vi "FRCts20_Backend_Test_Team.vi"() -> ()   [LabVIEW 2013, in "FRCts20_Backend_TestCode.lvlib"]
uses:
  FRCts20_Backend_TestCode.lvlib
  FRCts20_Backend_API/FRCts20_Backend_API_Command_App.ctl
  FRCts20_Backend_API/FRCts20_Backend_API_TeamRoot.ctl
  FRCts20_Backend_API/FRCts20_Backend_API_SW.ctl
  FRCts20_Backend_API/FRCts20_Backend_API_Team.ctl
  FRCts20_Backend_API/FRCts20_Backend_API_Status.ctl
  FRCts20_Backend_API/FRCts20_Backend_API_Application.vi
  FRCts20_Backend_API/FRCts20_Backend_API.lvlib
  FRCts20_Backend_Engine.lvlib
panel:
  out "Get Root Pass/Fail":bool
  out "Get Root":u32
  out "Get Pass/Fail":bool
  out "error out":errorcluster
  out "Del Pass/Fail":bool
  out "GetDel":u32
  out "Del":u32
  out "GetPut":u32
  out "Put":u32
  out "Put Pass/Fail":bool
  out "Post Pass/Fail":bool
  out "GetRootPost":u32
  out "post":u32
  out "Get":u32
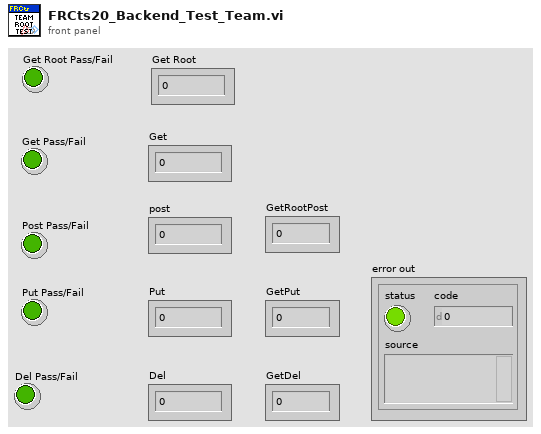
[diagram p1: front panel]
types:
  T1 = typedef "FRCts20_Backend_API.lvlib/FRCts20_Backend_API_Team.ctl" = cluster{"Team Index":u32, "Team Number":u32, "Team Name":string, "Short Team Name":string, "Nick Name":string, "Robot Name":string, "City":string, "State":string, "Country":string, "Rookie Year":u32, "SWType":T2, "CAN":bool, "Vision":bool, "Kinect":bool, "Tags":string, "Avatar":string, "Request Array":cluster{"Request Index":u32, "Description":string, "Status":T3, "Open Date":timestamp, "Last Update":timestamp, "Close Date":timestamp}[], "Events Attending":cluster{"EventIndex":dbl, "EventName":string, "IsLive":bool}[], "APIReturn":string}
  T2 = typedef "FRCts20_Backend_API.lvlib/FRCts20_Backend_API_SW.ctl" = string
  T3 = typedef "FRCts20_Backend_API.lvlib/FRCts20_Backend_API_Status.ctl" = enum16{"Open", "In Work", "Closed"}
  T4 = typedef "FRCts20_Backend_API.lvlib/FRCts20_Backend_API_TeamRoot.ctl" = cluster{"Teams":cluster{"Team Index":u32, "Team Number":u32, "Team Name":string, "Short Team Name":string, "Nick Name":string, "Robot Name":string, "City":string, "State":string, "Country":string, "Rookie Year":u32, "SWType":T2, "CAN":bool, "Vision":bool, "Kinect":bool, "Tags":string, "Avatar":string, "Events":cluster{"EventIndex":u32, "EventName":string, "IsLive":bool}[]}[], "APIReturn":string}
  T5 = typedef "FRCts20_Backend_API.lvlib/FRCts20_Backend_API_Command_App.ctl" = string
  T6 = cluster{"Team Index":u32, "Team Number":u32, "Team Name":string, "Short Team Name":string, "Nick Name":string, "Robot Name":string, "City":string, "State":string, "Country":string, "Rookie Year":u32, "SWType":T2, "CAN":bool, "Vision":bool, "Kinect":bool, "Tags":string, "Avatar":string, "Events":cluster{"EventIndex":u32, "EventName":string, "IsLive":bool}[]}[]
  T7 = cluster{"Team Index":u32, "Team Number":u32, "Team Name":string, "Short Team Name":string, "Nick Name":string, "Robot Name":string, "City":string, "State":string, "Country":string, "Rookie Year":u32, "SWType":T2, "CAN":bool, "Vision":bool, "Kinect":bool, "Tags":string, "Avatar":string, "Events":cluster{"EventIndex":u32, "EventName":string, "IsLive":bool}[]}
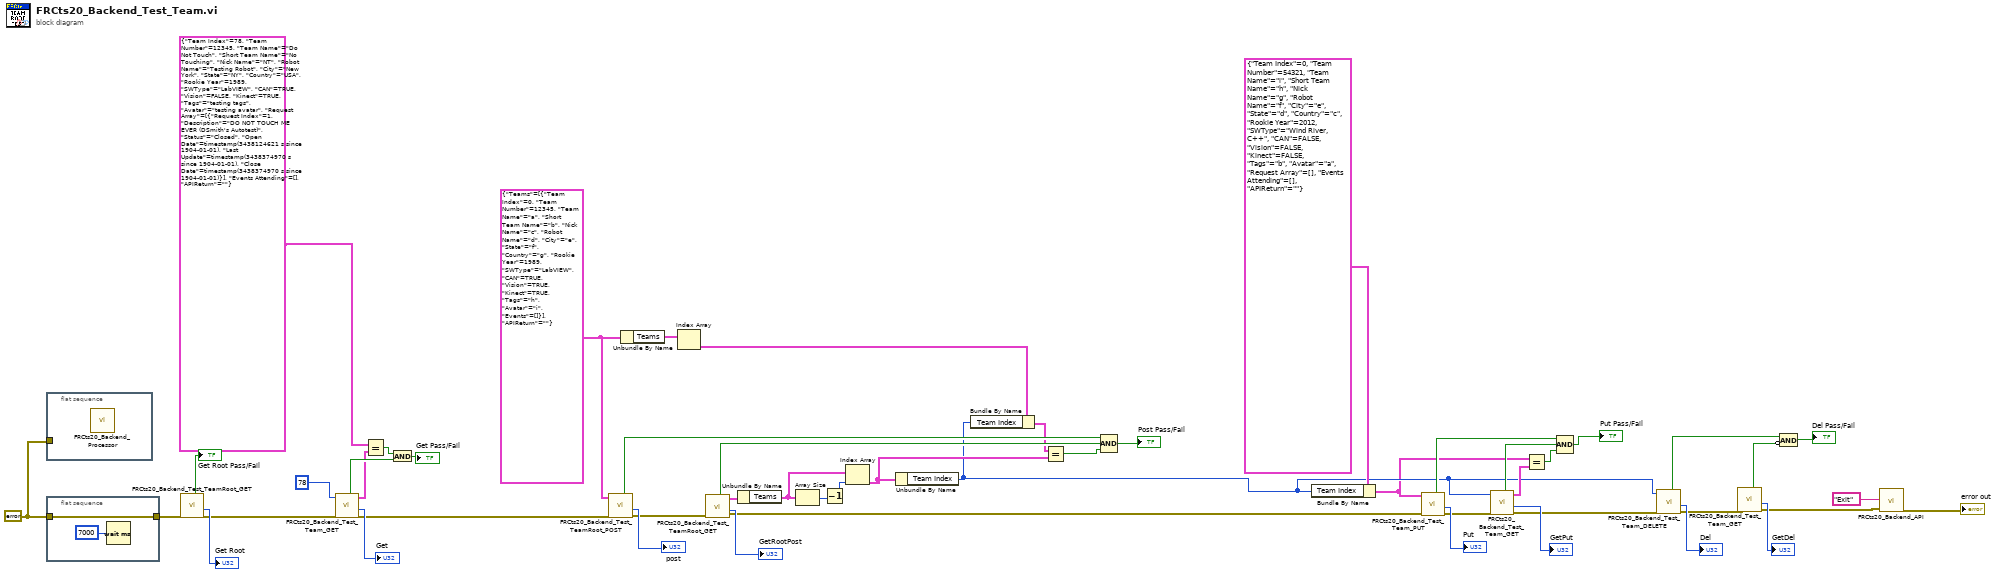
[diagram p0: block diagram]
diagram:
  w11 = T4 {"Teams"=[{"Team Index"=0, "Team Number"=12345, "Team Name"="a", "Short Team Name"="b", "Nick Name"="c", "Robot Name"="d", "City"="e", "State"="f", "Country"="g", "Rookie Year"=1989, "SWType"="LabVIEW", "CAN"=TRUE, "Vision"=TRUE, "Kinect"=TRUE, "Tags"="h", "Avatar"="i", "Events"=[]}], "APIReturn"=""} ("TeamRoot In")
  w50 = errorcluster {"status"=FALSE, "code"=0, "source"=""} ("error constant")
  n1 = flat-sequence {
    tunnel: w50 -> [_]
    frame #0 {
      n2 = call "FRCts20_Backend_Processor.vi"() -> ()  [unwired: 12 in]
    }
  }
  n3 = flat-sequence {
    tunnel: w50 -> [w52]
    tunnel: [w52] -> w48
    frame #0 {
      n4 = Wait (ms)(milliseconds to wait=u32 7000) -> ()  [unwired: 1 out]
    }
  }
  n5 = call "FRCts20_Backend_Test_TeamRoot_GET.vi"("error in (no error)"=w48) -> ("error out"=w45:errorcluster, "Time (ms)"=→"Get Root":u32, "Success"=→"Get Root Pass/Fail":bool)  [unwired: 6 in, 2 out]
  n6 = call "FRCts20_Backend_Test_Team_GET.vi"("error in (no error)"=w45, "Team Index"=u32 78) -> ("error out"=w42:errorcluster, "Time (ms)"=→"Get":u32, "Team Out"=w16:T1, "Success"=w18:bool)  [unwired: 5 in, 1 out]
  n7 = Equal?(x=T1 {"Team Index"=78, "Team Number"=12345, "Team Name"="Do Not Touch", "Short Team Name"="No Touching", "Nick Name"="NT", "Robot Name"="Testing Robot", "City"="New York", "State"="NY", "Country"="USA", "Rookie Year"=1989, "SWType"="LabVIEW", "CAN"=TRUE, "Vision"=FALSE, "Kinect"=TRUE, "Tags"="testing tags", "Avatar"="testing avatar", "Request Array"=[{"Request Index"=1, "Description"="DO NOT TOUCH ME EVER (DSmith's Autotest)", "Status"=enum."Closed", "Open Date"=timestamp(3438124621 s since 1904-01-01), "Last Update"=timestamp(3438374970 s since 1904-01-01), "Close Date"=timestamp(3438374970 s since 1904-01-01)}], "Events Attending"=[], "APIReturn"=""} ("Team Out"), y=w16) -> (x = y?=w17:bool)
  n8 = And(x=w17, y=w18) -> (x .and. y?=→"Get Pass/Fail":bool)
  n9 = call "FRCts20_Backend_Test_TeamRoot_POST.vi"("error in (no error)"=w42, "TeamRoot In"=w11) -> ("error out"=w40:errorcluster, "Time (ms)"=→"post":u32, "Success"=w29:bool)  [unwired: 5 in, 2 out]
  n10 = Unbundle By Name(w11) -> ("Teams"=w10:T6)
  n11 = Index Array(array=w10) -> (element=w8:T7)  [unwired: 1 in]
  n12 = call "FRCts20_Backend_Test_TeamRoot_GET.vi"("error in (no error)"=w40) -> ("error out"=w38:errorcluster, "Time (ms)"=→"GetRootPost":u32, "Team Out"=w15:T4, "Success"=w28:bool)  [unwired: 6 in, 1 out]
  n13 = Unbundle By Name(w15) -> ("Teams"=w12:T6)
  n14 = Array Size(array=w12) -> (size(s)=w14:i32)
  n15 = Decrement(x=w14) -> (x-1=w13:i32)
  n16 = Index Array(array=w12, index=w13) -> (element=w9:T7)
  n17 = Unbundle By Name(w9) -> ("Team Index"=w7:u32)
  n18 = Bundle By Name(cluster=w8, "Team Index"=w7) -> (w6:T7)
  n19 = Equal?(x=w6, y=w9) -> (x = y?=w27:bool)
  n20 = Compound Arithmetic op=AND(w29, w28, w27) -> (→"Post Pass/Fail":bool)
  n21 = Bundle By Name(cluster=T1 {"Team Index"=0, "Team Number"=54321, "Team Name"="i", "Short Team Name"="h", "Nick Name"="g", "Robot Name"="f", "City"="e", "State"="d", "Country"="c", "Rookie Year"=2012, "SWType"="Wind River, C++", "CAN"=FALSE, "Vision"=FALSE, "Kinect"=FALSE, "Tags"="b", "Avatar"="a", "Request Array"=[], "Events Attending"=[], "APIReturn"=""} ("Team In"), "Team Index"=w7) -> (w5:T1)
  n22 = call "FRCts20_Backend_Test_Team_PUT.vi"("error in (no error)"=w38, "Team In"=w5) -> ("error out"=w36:errorcluster, "Time (ms)"=→"Put":u32, "Success"=w24:bool)  [unwired: 5 in, 2 out]
  n23 = call "FRCts20_Backend_Test_Team_GET.vi"("error in (no error)"=w36, "Team Index"=w7) -> ("error out"=w34:errorcluster, "Time (ms)"=→"GetPut":u32, "Team Out"=w21:T1, "Success"=w23:bool)  [unwired: 5 in, 1 out]
  n24 = Equal?(x=w5, y=w21) -> (x = y?=w22:bool)
  n25 = Compound Arithmetic op=AND(w24, w23, w22) -> (→"Put Pass/Fail":bool)
  n26 = call "FRCts20_Backend_Test_Team_DELETE.vi"("error in (no error)"=w34, "Team Index"=w7) -> ("error out"=w32:errorcluster, "Time (ms)"=→"Del":u32, "Success"=w4:bool)  [unwired: 5 in, 2 out]
  n27 = call "FRCts20_Backend_Test_Team_GET.vi"("error in (no error)"=w32) -> ("error out"=w30:errorcluster, "Time (ms)"=→"GetDel":u32, "Success"=w3:bool)  [unwired: 6 in, 2 out]
  n28 = Compound Arithmetic op=AND(w4, invert w3) -> (→"Del Pass/Fail":bool)
  n29 = call-poly "FRCts20_Backend_API.vi"("error in (no error)"=w30, "Command"=T5 "Exit") -> ("error out"=→"error out":errorcluster)  [unwired: 7 in, 2 out]
